vi "ToRepo.vi"(8 "error in":errorcluster, 9 "to repo cluster":T1, 10 "repository in":refnum<class "NISE_CEF_Repository.lvclass">, 11 "node in":refnum<class "Targets.lvclass">) -> (0 "error out":errorcluster, 2 "repository out":refnum<class "NISE_CEF_Repository.lvclass">, 3 "node out":refnum<class "Targets.lvclass">)   [LabVIEW 2013, in "PL Framework Configuration Tool.lvlib" / "Targets.lvclass"]
doc: "Transfers the information from the tree node into the repo. How it is stored in the repo depends on the Repo."
uses:
  Targets.lvclass
  <vilib>/NI/Configuration Framework/Repository/NISE_CEF_Repository.lvclass
  <vilib>/NI/Configuration Framework/Node/ToRepoCluster.ctl
  Targets.lvclass/Targets.ctl
  TBM Configuration Node/TBM Configuration Node.lvclass
  <vilib>/NI/Configuration Framework/serializable configuration/NISE_CEF_serializable configuration.lvclass
  <vilib>/NI/Configuration Framework/Node/NISE_CEF_Node.lvclass
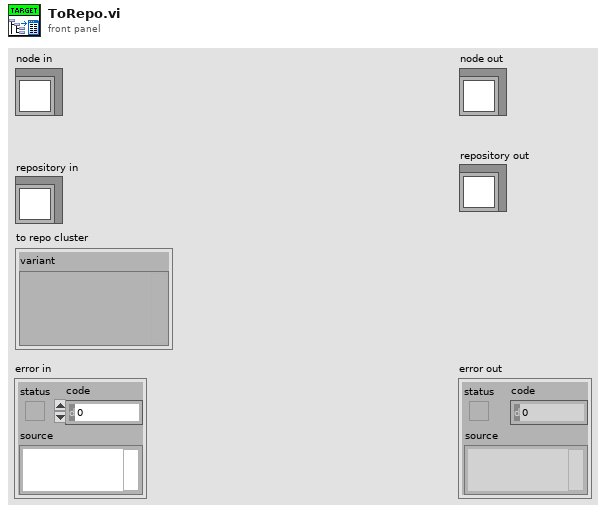
[diagram p1: front panel]
types:
  T1 = typedef "NISE_CEF_Node.lvclass/ToRepoCluster.ctl" = cluster{"variant":variant}
  T2 = typedef "PL Framework Configuration Tool.lvlib/TBM Configuration Node.lvclass/deployment configuration.ctl" = cluster{"local path":path, "remote path (relative to root)":path}
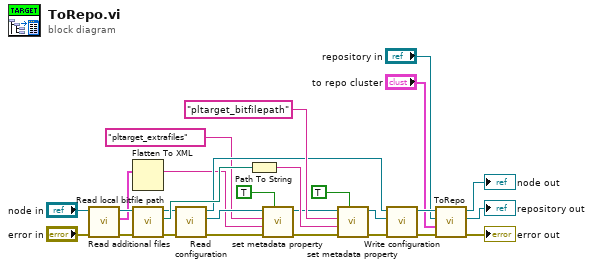
[diagram p0: block diagram]
diagram:
  n1 = call "Read additional files.vi"("error in"="error in", "Targets in"="node in") -> ("error out"=w9:errorcluster, "additional files"=w8:T2[], "Targets out"=w10:refnum<class "Targets.lvclass">)  [unwired: 7 in]
  n2 = Flatten To XML(anything=w8) -> (xml string=w2:string)
  n3 = call "Read local bitfile path.vi"("error in"=w9, "Targets in"=w10) -> ("error out"=w25:errorcluster, "bitfile path"=w22:path, "Targets out"=w19:refnum<class "Targets.lvclass">)  [unwired: 7 in]
  n4 = call-dynamic "Read configuration.vi"("error in"=w25, "NISE_CEF_serializable node in"=w19) -> ("error out"=w6:errorcluster, "configuration"=w7:refnum<class "NISE_CEF_serializable configuration.lvclass">, "NISE_CEF_serializable node out"=w17:refnum<class "Targets.lvclass">)  [unwired: 7 in]
  n5 = Path To String(path=w22) -> (string=w21:string)
  n6 = call <vilib>:"set metadata property.vi"("overwrite?"=TRUE, "error in"=w6, "value"=w2, "key"="pltarget_extrafiles", "configuration in"=w7) -> ("error out"=w1:errorcluster, "configuration out"=w5:refnum<class "NISE_CEF_serializable configuration.lvclass">)  [unwired: 5 in]
  n7 = call <vilib>:"set metadata property.vi"("overwrite?"=TRUE, "error in"=w1, "value"=w21, "key"="pltarget_bitfilepath", "configuration in"=w5) -> ("error out"=w24:errorcluster, "configuration out"=w15:refnum<class "NISE_CEF_serializable configuration.lvclass">)  [unwired: 5 in]
  n8 = call-dynamic "Write configuration.vi"("error in"=w24, "configuration"=w15, "NISE_CEF_serializable node in"=w17) -> ("error out"=w18:errorcluster, "NISE_CEF_serializable node out"=w16:refnum<class "Targets.lvclass">)  [unwired: 7 in]
  n9 = call-parent "ToRepo.vi"("error in"=w18, "to repo cluster"="to repo cluster", "repository in"="repository in", "node in"=w16) -> ("error out"=→"error out":errorcluster, "repository out"=→"repository out":refnum<class "NISE_CEF_Repository.lvclass">, "node out"=→"node out":refnum<class "Targets.lvclass">)  [unwired: 5 in]
